vi "Create Message Status.vi"(8 "error in (no error)":errorcluster, 10 "Channel Paramters":T2, 11 "Message Channels Section in":T1 format="%.0x") -> (0 "error out":errorcluster, 3 "Message Channels Section out":T1 format="%.0x")   [LabVIEW 2020, in "Instrument Addon Scripting API.lvlib"]
uses:
  Instrument Addon Scripting API.lvlib
  <vilib>/NI VeriStand/Custom Device API/Custom Device Item Ref.ctl
  <vilib>/NI VeriStand/Custom Device API/Custom Device Channel.ctl
  <vilib>/NI VeriStand/Custom Device API/Custom Device Channel Type.ctl
  Shared Directory/Constants.vi
  Shared Directory/Instrument Addon Shared.lvlib
  <vilib>/NI VeriStand/Custom Device API/Custom Device API.lvlib
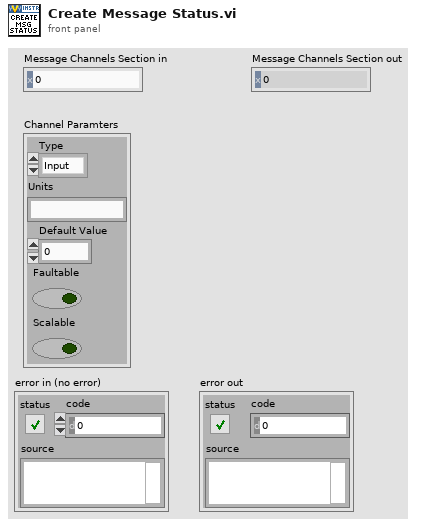
[diagram p1: front panel]
types:
  T1 = typedef "Custom Device API.lvlib/Custom Device Item Ref.ctl" = u64
  T2 = typedef "Custom Device API.lvlib/Custom Device Channel.ctl" = cluster{"Type":T3, "Units":string, "Default Value":dbl, "Faultable":bool, "Scalable":bool}
  T3 = typedef "Custom Device API.lvlib/Custom Device Channel Type.ctl" = enum16{"Input", "Output"}
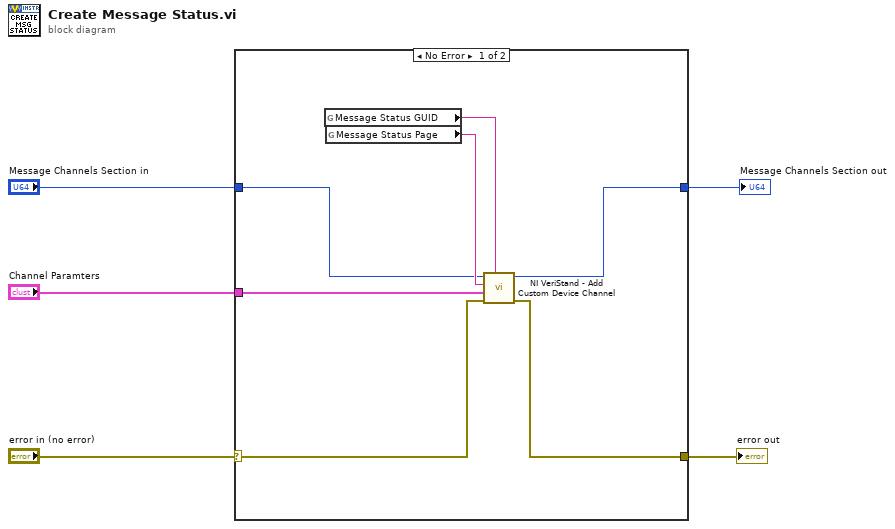
[diagram p0: block diagram]
diagram:
  n1 = case shown="No Error" "error in (no error)" {
    selector: "error in (no error)" -> [w6 w13]
    tunnel: [w10 w14] -> w5
    tunnel: [w9 w13] -> w4
    tunnel: "Channel Paramters" -> [w8 _]
    tunnel: "Message Channels Section in" -> [w7 w14]
    frame No Error {
      n2 = global read "Constants.vi" "Message Status GUID"() -> (w11:string)
      n3 = global read "Constants.vi" "Message Status Page"() -> (w12:string)
      n4 = call <vilib>:"NI VeriStand - Add Custom Device Channel.vi"("GUID (Default Channel)"=w11, "error in (no error)"=w6, "Channel"=w8, "Channel Name"=w12, "Parent Ref in"=w7) -> ("error out"=w9:errorcluster, "Parent Ref out"=w10:T1)  [unwired: 3 in, 2 out]
    }
    frame Error {
    }
  }
  "Message Channels Section out" <- w5
  "error out" <- w4
